vi "fpga_start.vi"(8 "error in":errorcluster, 9 "Bit rate":dbl=400000.0 format="%#_6p", 11 "I2C interface":T1) -> (0 "error out":errorcluster)   [LabVIEW 2013]
uses:
  i2c_interface.ctl
  fpga_reference.ctl
  i2c_defs.vi
  asap/labview/initialization/globals.vi
  <vilib>/Utility/error.llb/Error Cluster From Error Code.vi
  <vilib>/rvi/errors/niLvFpgaAdjustHostInterfaceError.vi
  <vilib>/FPGAPlugInAG/PCIe-7842R/niLvFpga_Run_PCIe-7842R.vi
  <vilib>/rvi/interface/nirviReadWriteControl/nirviReadWriteControl.xnode
  FPGA Bitfiles/i2cmuxdemux.lvbitx
  <vilib>/rvi/interface/nirviMethod/nirviMethod.xnode
  NiFpgaLv.dll
panel:
  # "Reset and start the FPGA.  This shouldn't be done until after all DAQ tasks triggered off of the FPGA have been started."
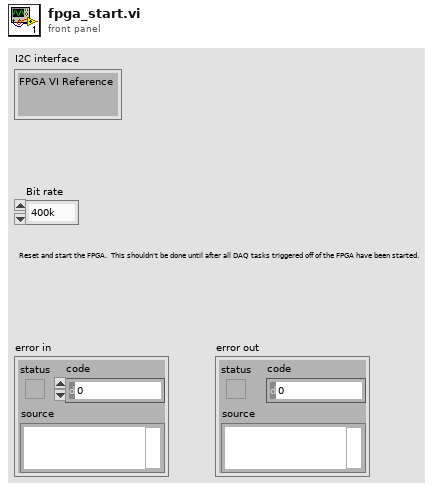
[diagram p1: front panel]
types:
  T1 = typedef "i2c_interface.ctl" = cluster{"FPGA VI Reference":T2}
  T2 = typedef "fpga_reference.ctl" = refnum<k20>
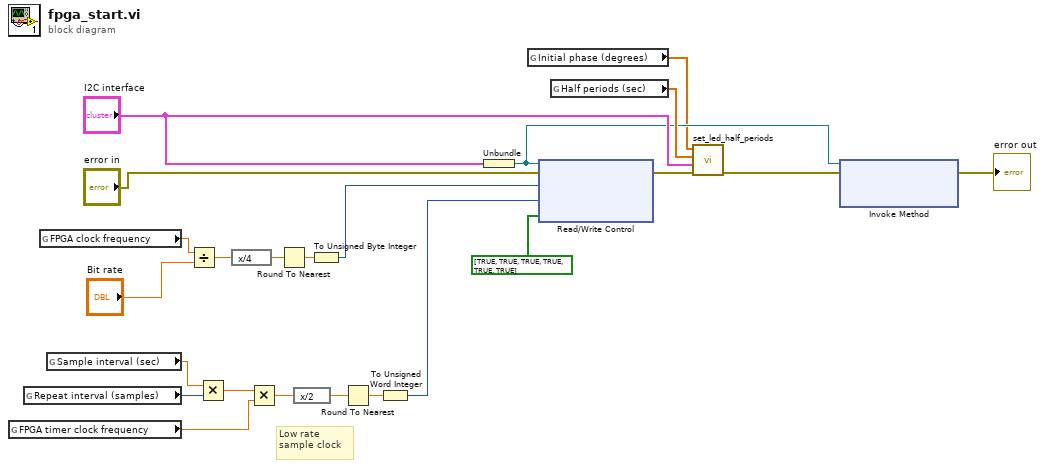
[diagram p0: block diagram]
diagram:
  # "Low rate sample clock"
  n1 = global read "i2c_defs.vi" "FPGA timer clock frequency"() -> (w5:dbl)
  n2 = global read "globals.vi" "Repeat interval (samples)"() -> (w8:i32)
  n3 = global read "i2c_defs.vi" "FPGA clock frequency"() -> (w18:dbl)
  n4 = global read "globals.vi" "Sample interval (sec)"() -> (w7:dbl)
  n5 = Divide(x=w18, y="Bit rate") -> (x/y=w21:dbl)
  n6 = Multiply(x=w7, y=w8) -> (x*y=w6:dbl)
  n7 = expression code="x/4"(w21) -> (w20:dbl)
  n8 = Multiply(x=w6, y=w5) -> (x*y=w4:dbl)
  n9 = Round To Nearest(number=w20) -> (nearest integer value=w19:dbl)
  n10 = expression code="x/2"(w4) -> (w3:dbl)
  n11 = To Unsigned Byte Integer(number=w19) -> (unsigned 8bit integer=w23:u8)
  n12 = Round To Nearest(number=w3) -> (nearest integer value=w2:dbl)
  n13 = To Unsigned Word Integer(number=w2) -> (unsigned 16bit integer=w1:u16)
  n14 = Unbundle("I2C interface") -> ("FPGA VI Reference"=w11:T2)
  n15 = global read "globals.vi" "Initial phase (degrees)"() -> (w9:dbl[])
  n16 = xnode "Read/Write Control"("FPGA VI Reference In"=w11, "error in"="error in", "I2C clock divisor"=w23, "Lo rate half period"=w1, "Output enable"=bool[] [TRUE, TRUE, TRUE, TRUE, TRUE, TRUE]) -> ("error out"=w15:errorcluster)  [unwired: 1 out]
  n17 = global read "globals.vi" "Half periods (sec)"() -> (w13:dbl[])
  n18 = call "set_led_half_periods.vi"("error in"=w15, "I2C interface"="I2C interface", "Half periods (sec)"=w13, "Initial phase (degrees)"=w9) -> ("error out"=w12:errorcluster)  [unwired: 7 in]
  n19 = xnode "Invoke Method"("FPGA VI Reference In"=w11, "error in"=w12) -> ("error out"=→"error out":errorcluster)  [unwired: 1 in, 1 out]
